vi "AI Init.vi"(7 "ADC #":T1=-1, 8 "error in (no error)":errorcluster, 11 "DeviceComms in":refnum<class "DeviceComms.lvclass">) -> (0 "error out":errorcluster, 3 "DeviceComms out":refnum<class "DeviceComms.lvclass">)   [LabVIEW 2020, in "CTI.lvlib" / "DeviceComms.lvclass"]
uses:
  DeviceComms.lvclass
  ADC Number.ctl
  CTI.lvlib
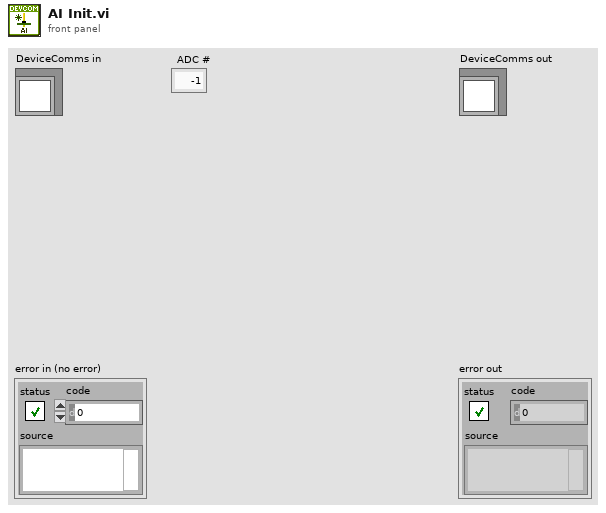
[diagram p1: front panel]
types:
  T1 = typedef "CTI.lvlib/ADC Number.ctl" = i8
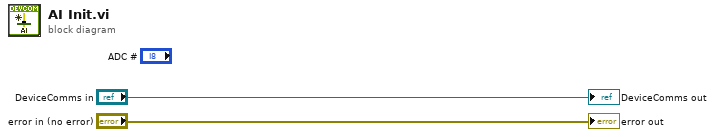
[diagram p0: block diagram]
diagram:
  "error out" <- "error in (no error)"
  "DeviceComms out" <- "DeviceComms in"
